vi "GE 5565PIORC.Memory.Write to DMA Block (DBL).vi"(8 "error in (no error)":errorcluster, 9 "data":dbl[](array[numeric]), 10 "Block Descriptor in":T1 {"next descriptor ptr" format="%08x"; "data size" format="%08x"; "data ptr (upper)" format="%08x"; "data ptr (lower)" format="%08x"; "descriptor ptr (aligned)" format="%08x"; "descriptor size" format="%08x"; "descriptor ptr (VISA)" format="%08x"}, 11 "GE 5565PIORC in":refnum<class "GE 5565PIORC.lvclass">) -> (0 "error out":errorcluster, 1 "data out":dbl[](array[numeric]), 2 "Block Descriptor out":T1 {"next descriptor ptr" format="%08x"; "data size" format="%08x"; "data ptr (upper)" format="%08x"; "data ptr (lower)" format="%08x"; "descriptor ptr (aligned)" format="%08x"; "descriptor size" format="%08x"; "descriptor ptr (VISA)" format="%08x"}, 3 "GE 5565PIORC out":refnum<class "GE 5565PIORC.lvclass">)   [LabVIEW 2016, in "GE 5565PIORC.lvclass"]
doc: "Writes the contents of the <B>data</B> array to the specified <B>Block Descriptor</B>. The number of elements transferred will be either the number of elements in <B>data</B> or a number of elements resulting in a size that is less than or equal to the allocated size of the <B>Block Descriptor</B>, whichever is smaller."
uses:
  GE 5565PIORC.lvclass
  Typedefs/GE 5565PIORC.Typdef.DMA Block Descriptor.ctl
  GE 5565PIORC.lvclass/GE 5565PIORC.ctl
  <vilib>/Instr/_visa.llb/VISA Register Access Address Space.ctl
  GE 5565PIORC.Memory.VISA Return Handler.vi
  <vilib>/Utility/error.llb/Error Cluster From Error Code.vi
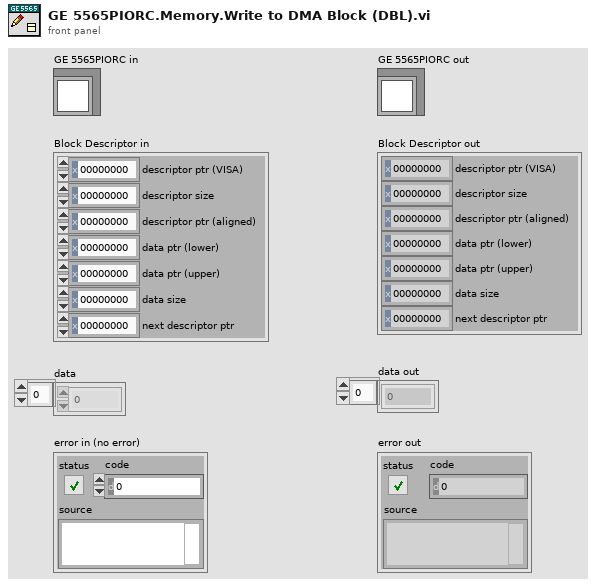
[diagram p1: front panel]
types:
  T1 = typedef "GE 5565PIORC.lvclass/GE 5565PIORC.Typdef.DMA Block Descriptor.ctl" = cluster{"descriptor ptr (VISA)":u32, "descriptor size":u32, "descriptor ptr (aligned)":u32, "data ptr (lower)":u32, "data ptr (upper)":u32, "data size":u32, "next descriptor ptr":u32}
  T2 = typedef "VISA Register Access Address Space.ctl" = u16
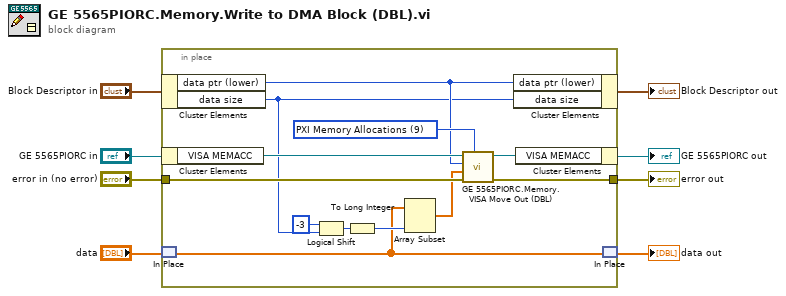
[diagram p0: block diagram]
diagram:
  n1 = in-place {
    in-place-border: "error in (no error)" -> [w20]
    in-place-border: [w19] -> w7
    w16 = T2 9 items=["VXI/VME A16"=1, "VXI/VME A24"=2, "VXI/VME A32"=3, "VXI/VME A64"=4, "PXI Memory Allocations"=9, "PXI Configuration"=10, "PXI BAR0"=11, "PXI BAR1"=12, "PXI BAR2"=13, "PXI BAR3"=14, "PXI BAR4"=15, "PXI BAR5"=16] ("address space")
    n2 = in-place-cluster #1("Block Descriptor in") -> ("data ptr (lower)"=w11:u32, "data size"=w9:u32)
    n3 = in-place-cluster #2("GE 5565PIORC in") -> ("VISA MEMACC"=w18:refnum<visa-resource-name>)
    n4 = in-place-match #3("data") -> (w10:dbl[])
    n5 = Logical Shift(y=i16 -3, x=w9) -> (x << y=w14:u32)
    n6 = To Long Integer(number=w14) -> (32bit integer=w13:i32)
    n7 = Array Subset(array=w10, length=w13) -> (w12:dbl[])  [unwired: 1 in]
    n8 = call "GE 5565PIORC.Memory.VISA Move Out (DBL).vi"("address space"=w16, "error in (no error)"=w20, "data"=w12, "offset (0)"=w11, "VISA resource name"=w18) -> ("error out"=w19:errorcluster, "VISA resource name out"=w17:refnum<visa-resource-name>)  [unwired: 5 in]
    n9 = in-place-cluster #1("data ptr (lower)"=w11, "data size"=w9) -> (→"Block Descriptor out":T1)
    n10 = in-place-cluster #2("VISA MEMACC"=w17) -> (→"GE 5565PIORC out":refnum<class "GE 5565PIORC.lvclass">)
    n11 = in-place-match #3(w10) -> (→"data out":dbl[])
  }
  "error out" <- w7
